vi "SRV_Init_Comm.vi"(8 "error in (no error)":errorcluster, 11 "SRV IP Address":string) -> (0 "error out":errorcluster, 1 "Cancelled?":bool, 2 "SRV IP Address out":string, 3 "connection ID":refnum<k5>)   [LabVIEW 2009]
doc: "Opens a session with the SRV.\n\n\nWritten for Benilde St. Margaret's School - Tim Jump\nBy Doug Schmertman - Logic PD\nCopyright 2012"
panel:
  # "This LabVIEW item is deprecated.\n\nIt is believed to be unused and will be removed in a future version of SRV."
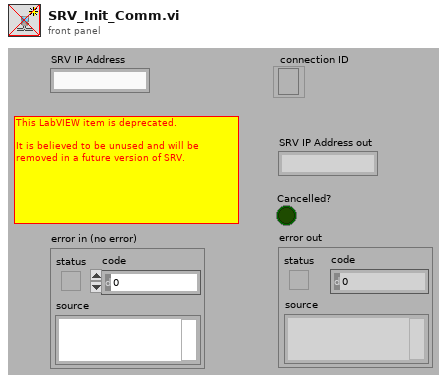
[diagram p1: front panel]
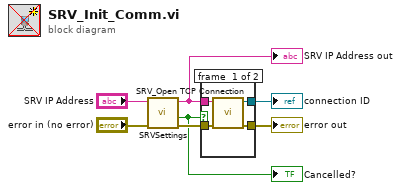
[diagram p0: block diagram]
diagram:
  n1 = call "SRVSettings.vi"("error in (no error)"="error in (no error)", "SRV IP Address"="SRV IP Address") -> ("error out"=w2:errorcluster, "Cancelled?"=w1:bool, "SRV IP Address out"=w4:string)  [unwired: 7 in]
  "SRV IP Address out" <- w4
  "Cancelled?" <- w1
  n2 = case shown="False" w1 {
    tunnel: [w11 _] -> w6
    tunnel: [w10 w12] -> w5
    tunnel: w4 -> [w9 _]
    tunnel: w2 -> [w8 w12]
    frame #0 {
      n3 = call "SRV_Open TCP Connection.vi"("error in (no error)"=w8, "IP address"=w9) -> ("error out"=w10:errorcluster, "connection ID"=w11:refnum<k5>)  [unwired: 8 in]
    }
    frame #1 {
    }
  }
  "connection ID" <- w6
  "error out" <- w5
